vi "main.vi"   [LabVIEW 2018]
uses:
  <vilib>/Instr/_visa.llb/VISA Configure Serial Port (Instr).vi
panel:
  # "主程序"
types:
  T1 = typedef "数据簇.ctl" = cluster{"字符串":string, "数值":i32, "布尔":bool}
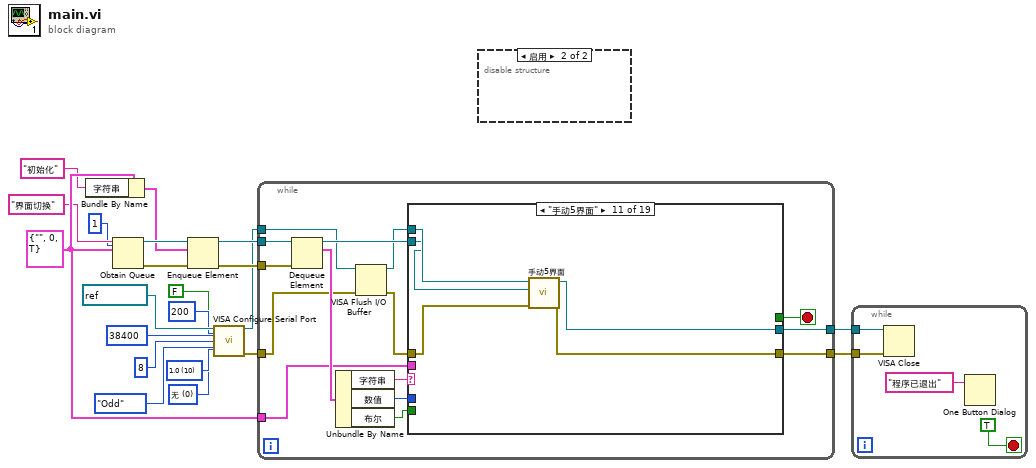
[diagram p0: block diagram]
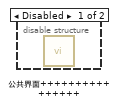
[diagram p2: hidden frame]
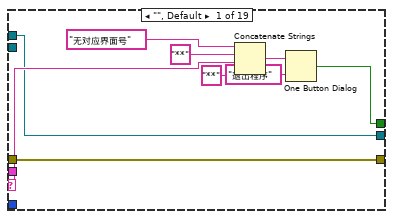
[diagram p3: hidden frame]
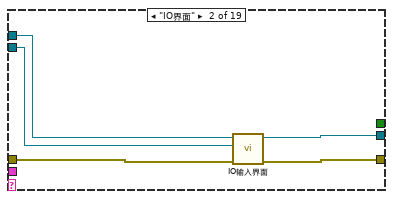
[diagram p4: hidden frame]
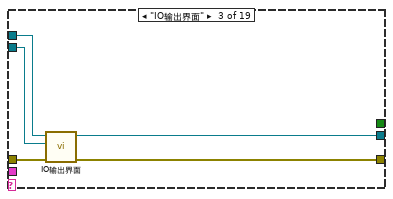
[diagram p5: hidden frame]
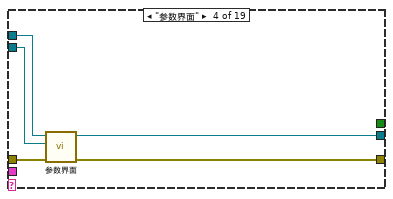
[diagram p6: hidden frame]
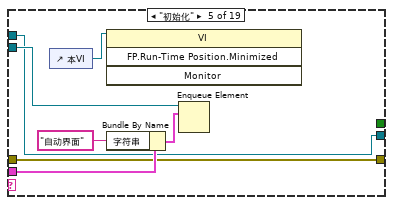
[diagram p7: hidden frame]
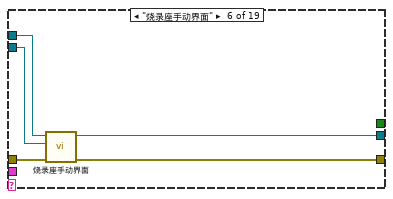
[diagram p8: hidden frame]
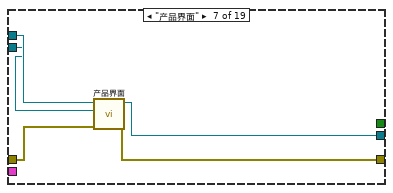
[diagram p9: hidden frame]
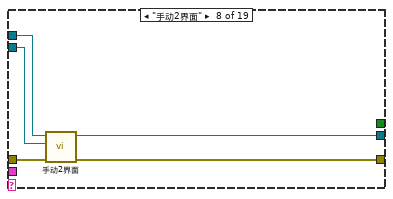
[diagram p10: hidden frame]
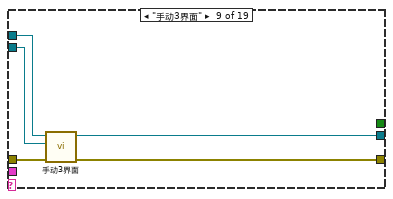
[diagram p11: hidden frame]
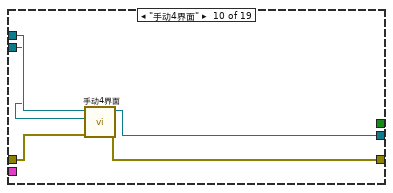
[diagram p12: hidden frame]
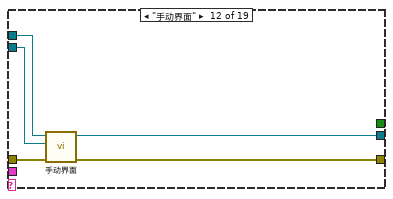
[diagram p13: hidden frame]
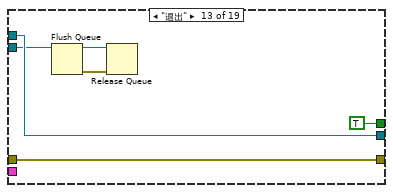
[diagram p14: hidden frame]
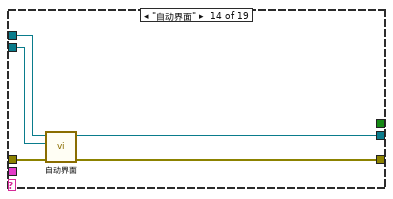
[diagram p15: hidden frame]
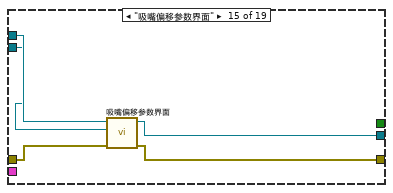
[diagram p16: hidden frame]
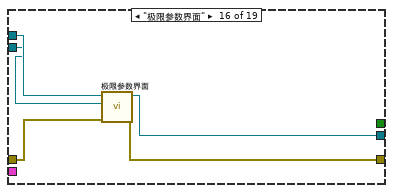
[diagram p17: hidden frame]
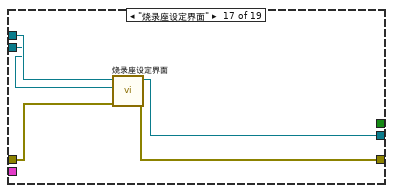
[diagram p18: hidden frame]
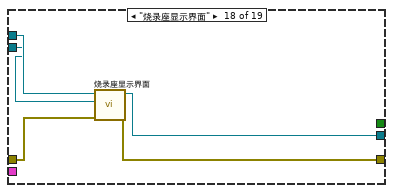
[diagram p19: hidden frame]
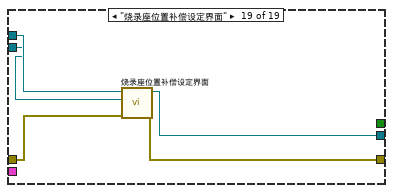
[diagram p20: hidden frame]
diagram:
  w2 = u16 0 items=["无", "XON/XOFF", "RTS/CTS", "XON/XOFF & RTS/CTS", "DTR/DSR", "XON/XOFF & DTR/DSR"] ("flow control (0:none)")
  w3 = u16 10 items=["1.0"=10, "1.5"=15, "2.0"=20] ("stop bits (10: 1 bit)")
  w19 = T1 {"字符串"="", "数值"=0, "布尔"=TRUE}
  n1 = Bundle By Name(cluster=w19, "字符串"="初始化") -> (w11:T1)
  n2 = Obtain Queue(max queue size (-1, unlimited)=1 ("队列最大值（-1，无限）"), name (unnamed)="界面切换" ("名称（未命名）"), element data type=w19) -> (queue out=w13:refnum<queue>, error out=w12:errorcluster)  [unwired: 2 in, 1 out]
  n3 = Enqueue Element(queue=w13, element=w11, error in (no error)=w12) -> (queue out=w21:refnum<queue>, error out=w20:errorcluster)  [unwired: 1 in, 1 out]
  n4 = call-poly "VISA Configure Serial Port"("VISA resource name"=refnum<visa-resource-name> "COM3", "timeout (10sec)"=u32 200, "Enable Termination\nChar (T)"=FALSE ("Enable Termination\nChar (T)"), "baud rate (9600)"=u32 38400, "data bits (8)"=u16 8, "parity (0:none)"=enum16{"None", "Odd", "Even", "Mark", "Space"}."Odd", "stop bits (10: 1 bit)"=w3, "flow control (0:none)"=w2) -> ("VISA resource name out"=w18:refnum<visa-resource-name>, "error out"=w17:errorcluster)  [unwired: 6 in]
  n5 = while {
    tunnel: w21 -> [w36]
    tunnel: w20 -> [w35]
    tunnel: w19 -> [w30]
    tunnel: w18 -> [w25]
    tunnel: w17 -> [w24]
    tunnel: [w29] -> w16
    tunnel: [w28] -> w15
    stop <- w33 stop-if-true
    n6 = Dequeue Element(queue=w36, error in (no error)=w35) -> (queue out=w34:refnum<queue>, element=w32:T1)  [unwired: 1 in, 2 out]
    n7 = Unbundle By Name(w32) -> ("字符串"=w31:string, "数值"=w27:i32, "布尔"=w26:bool)
    n8 = VISA Flush I/O Buffer(VISA resource name=w25, error in (no error)=w24) -> (VISA resource name out=w23:refnum<visa-resource-name>, error out=w22:errorcluster)  [unwired: 1 in]
    n9 = case shown="\"手动5界面\"" w31 {
      selector: w31 -> [w43 _ _ _ _ _ _ _ _ _ _ _ _ _ _ _ _ _ _]
      tunnel: w34 -> [_ w46 w53 w56 w67 w70 w76 w80 w85 w90 w96 w98 w105 w109 w117 w122 w127 w132 w137]
      tunnel: [w38 _ _ _ _ _ _ _ _ _ _ _ TRUE _ _ _ _ _ _] -> w33
      tunnel: w30 -> [_ _ _ _ w65 _ _ _ _ _ _ _ _ _ _ _ _ _ _]
      tunnel: w23 -> [w40 w50 w55 w60 w62 w72 w77 w82 w87 w92 w97 w102 w107 w113 w118 w123 w128 w133 w138]
      tunnel: w22 -> [w39 w49 w54 w59 w61 w71 w75 w81 w86 w91 w95 w99 w106 w112 w116 w121 w126 w131 w136]
      tunnel: [w40 w48 w52 w58 w62 w69 w74 w79 w84 w89 w94 w101 w107 w111 w115 w120 w125 w130 w135] -> w29
      tunnel: [w39 w47 w51 w57 w61 w68 w73 w78 w83 w88 w93 w100 w106 w110 w114 w119 w124 w129 w134] -> w28
      tunnel: w27 -> [_ _ _ _ _ _ _ _ _ _ _ _ _ _ _ _ _ _ _]
      tunnel: w26 -> [_ _ _ _ _ _ _ _ _ _ _ _ _ _ _ _ _ _ _]
      frame "", Default {
        n10 = Concatenate Strings("无对应界面号" ("消息"), "**" ("字符串"), w43, "**" ("字符串")) -> (w41:string)
        n11 = One Button Dialog(message=w41, button name ("OK")="退出程序" ("按钮名称（“确定”）")) -> (true=w38:bool)
      }
      frame "IO界面" {
        n12 = call "IO输入界面.vi"("错误输入（无错误）"=w49, "界面切换队列"=w46, "VISA资源名称输入"=w50) -> ("错误输出"=w47:errorcluster, "VISA资源名称输出"=w48:refnum<visa-resource-name>)  [unwired: 7 in]
      }
      frame "IO输出界面" {
        n13 = call "IO输出界面.vi"("错误输入（无错误）"=w54, "界面切换队列"=w53, "VISA资源名称输入"=w55) -> ("错误输出"=w51:errorcluster, "VISA资源名称输出"=w52:refnum<visa-resource-name>)  [unwired: 7 in]
      }
      frame "参数界面" {
        n14 = call "参数界面.vi"("错误输入（无错误）"=w59, "界面切换队列"=w56, "VISA资源名称输入"=w60) -> ("错误输出"=w57:errorcluster, "VISA资源名称输出"=w58:refnum<visa-resource-name>)  [unwired: 7 in]
      }
      frame "初始化" {
        n15 = control-ref of="本VI"() -> (w66:refnum<vi>)
        n16 = invoke class="VI" method="FP.Run-Time Position.Minimized"(reference=w66) -> ()  [unwired: 3 in, 4 out]
        n17 = Bundle By Name(cluster=w65, "字符串"="自动界面") -> (w63:T1)
        n18 = Enqueue Element(queue=w67, element=w63) -> ()  [unwired: 2 in, 3 out]
      }
      frame "烧录座手动界面" {
        n19 = call "烧录座手动界面.vi"("错误输入（无错误）"=w71, "界面切换队列"=w70, "VISA资源名称输入"=w72) -> ("错误输出"=w68:errorcluster, "VISA资源名称输出"=w69:refnum<visa-resource-name>)  [unwired: 7 in]
      }
      frame "产品界面" {
        n20 = call "产品界面.vi"("错误输入（无错误）"=w75, "界面切换队列"=w76, "VISA资源名称输入"=w77) -> ("错误输出"=w73:errorcluster, "VISA资源名称输出"=w74:refnum<visa-resource-name>)  [unwired: 7 in]
      }
      frame "手动2界面" {
        n21 = call "手动2界面.vi"("错误输入（无错误）"=w81, "界面切换队列"=w80, "VISA资源名称输入"=w82) -> ("错误输出"=w78:errorcluster, "VISA资源名称输出"=w79:refnum<visa-resource-name>)  [unwired: 7 in]
      }
      frame "手动3界面" {
        n22 = call "手动3界面.vi"("错误输入（无错误）"=w86, "界面切换队列"=w85, "VISA资源名称输入"=w87) -> ("错误输出"=w83:errorcluster, "VISA资源名称输出"=w84:refnum<visa-resource-name>)  [unwired: 7 in]
      }
      frame "手动4界面" {
        n23 = call "手动4界面.vi"("错误输入（无错误）"=w91, "界面切换队列"=w90, "VISA资源名称输入"=w92) -> ("错误输出"=w88:errorcluster, "VISA资源名称输出"=w89:refnum<visa-resource-name>)  [unwired: 7 in]
      }
      frame "手动5界面" {
        n24 = call "手动5界面.vi"("错误输入（无错误）"=w95, "界面切换队列"=w96, "VISA资源名称输入"=w97) -> ("错误输出"=w93:errorcluster, "VISA资源名称输出"=w94:refnum<visa-resource-name>)  [unwired: 7 in]
      }
      frame "手动界面" {
        n25 = call "手动界面.vi"("错误输入（无错误）"=w99, "界面切换队列"=w98, "VISA资源名称输入"=w102) -> ("错误输出"=w100:errorcluster, "VISA资源名称输出"=w101:refnum<visa-resource-name>)  [unwired: 7 in]
      }
      frame "退出" {
        n26 = Flush Queue(queue=w105) -> (queue out=w104:refnum<queue>, error out=w103:errorcluster)  [unwired: 1 in, 1 out]
        n27 = Release Queue(queue=w104, error in (no error)=w103) -> ()  [unwired: 1 in, 3 out]
      }
      frame "自动界面" {
        n28 = call "自动界面.vi"("错误输入（无错误）"=w112, "界面切换队列"=w109, "VISA资源名称输入"=w113) -> ("错误输出"=w110:errorcluster, "VISA资源名称输出"=w111:refnum<visa-resource-name>)  [unwired: 7 in]
      }
      frame "吸嘴偏移参数界面" {
        n29 = call "吸嘴偏移参数界面.vi"("错误输入（无错误）"=w116, "界面切换队列"=w117, "VISA资源名称输入"=w118) -> ("错误输出"=w114:errorcluster, "VISA资源名称输出"=w115:refnum<visa-resource-name>)  [unwired: 7 in]
      }
      frame "极限参数界面" {
        n30 = call "极限参数界面.vi"("错误输入（无错误）"=w121, "界面切换队列"=w122, "VISA资源名称输入"=w123) -> ("错误输出"=w119:errorcluster, "VISA资源名称输出"=w120:refnum<visa-resource-name>)  [unwired: 7 in]
      }
      frame "烧录座设定界面" {
        n31 = call "烧录座设定界面.vi"("错误输入（无错误）"=w126, "界面切换队列"=w127, "VISA资源名称输入"=w128) -> ("错误输出"=w124:errorcluster, "VISA资源名称输出"=w125:refnum<visa-resource-name>)  [unwired: 7 in]
      }
      frame "烧录座显示界面" {
        n32 = call "烧录座显示界面.vi"("错误输入（无错误）"=w131, "界面切换队列"=w132, "VISA资源名称输入"=w133) -> ("错误输出"=w129:errorcluster, "VISA资源名称输出"=w130:refnum<visa-resource-name>)  [unwired: 7 in]
      }
      frame "烧录座位置补偿设定界面" {
        n33 = call "烧录座位置补偿设定界面.vi"("错误输入（无错误）"=w136, "界面切换队列"=w137, "VISA资源名称输入"=w138) -> ("错误输出"=w134:errorcluster, "VISA资源名称输出"=w135:refnum<visa-resource-name>)  [unwired: 7 in]
      }
    }
  }
  n34 = disable-structure shown="启用" {
    frame Disabled {
      n35 = call "公共界面++++++++++++++++.vi"() -> ()  [unwired: 10 in, 2 out]
    }
    frame Enabled {
    }
  }
  n36 = while {
    tunnel: w16 -> [w142]
    tunnel: w15 -> [w141]
    stop <- TRUE stop-if-true
    n37 = VISA Close(VISA resource name=w142, error in (no error)=w141) -> ()  [unwired: 1 out]
    n38 = One Button Dialog(message="程序已退出" ("消息")) -> ()  [unwired: 1 in, 1 out]
  }
